vi "Count Digital Pulses Get Date.vi"() -> ()   [LabVIEW 2020]
uses:
  <vilib>/DAQmx/read.llb/DAQmx Read (Counter U32 1Chan 1Samp).vi
  <vilib>/DAQmx/create/channels.llb/DAQmx Create Channel (CI-Count Edges).vi
  <vilib>/DAQmx/miscellaneous.llb/DAQmx Fill In Error Info.vi
panel:
  out "Frequency (Hz)":dbl
  in  "stop":bool
  out "Counts":dbl
  in  "edge":i32(ring)=10280 items=["Rising"=10280, "Falling"=10171]
  in  "count direction":i32(ring)=10128 items=["Count Up"=10128, "Count Down"=10124, "Externally Controlled"=10326]
  in  "initial count":u32
  in  "DAQmx Physical Channel":tag
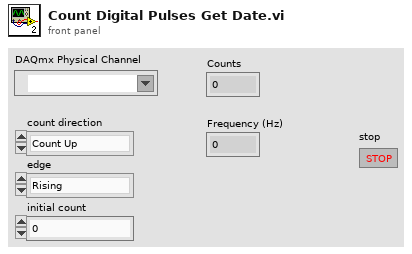
[diagram p1: front panel]
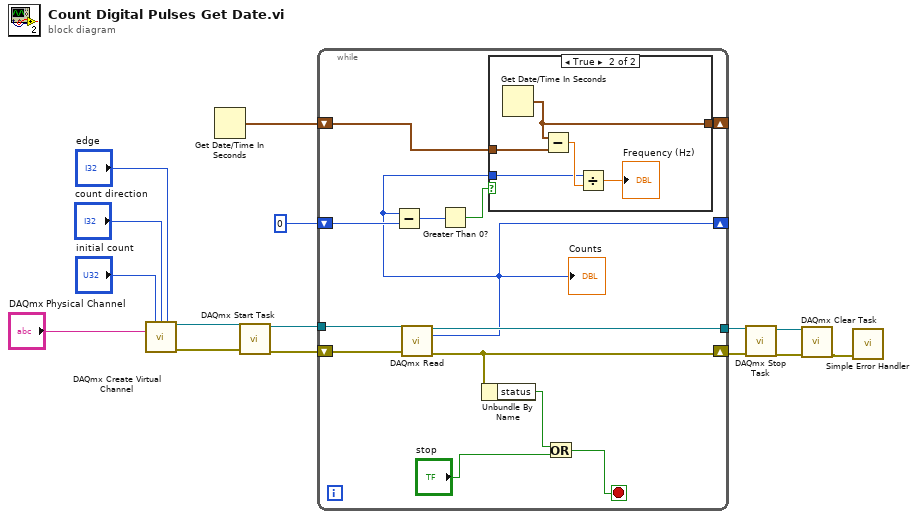
[diagram p0: block diagram]
diagram:
  n1 = call-poly <vilib>:"DAQmx Create Virtual Channel.vi"("initial count"="initial count", "count direction"="count direction", "edge"="edge", "counter"="DAQmx Physical Channel") -> ("task out"=w12:refnum<k21>, "error out"=w11:errorcluster)  [unwired: 10 in]
  n2 = Get Date/Time In Seconds() -> (seconds since 1Jan1904=w1:timestamp)
  n3 = call <vilib>:"DAQmx Start Task.vi"("task/channels in"=w12, "error in"=w11) -> ("task out"=w10:refnum<k21>, "error out"=w9:errorcluster)  [unwired: 12 in]
  n4 = while {
    tunnel: w10 -> [w28]
    tunnel: [w26] -> w8
    shift-right: [w25] -> w7
    shift-left: w9 -> [w27]
    shift-right: [w16] -> _
    shift-left: 0 -> [w21]
    shift-right: [w17] -> _
    shift-left: w1 -> [w18]
    stop <- w22 stop-if-true
    n5 = call-poly <vilib>:"DAQmx Read.vi"("task/channels in"=w28, "error in"=w27) -> ("task out"=w26:refnum<k21>, "data"=w16:u32, "error out"=w25:errorcluster)  [unwired: 11 in]
    "Counts" <- w16
    n6 = Subtract(x=w16, y=w21) -> (x-y=w20:u32)
    n7 = Greater Than 0?(x=w20) -> (x > 0?=w19:bool)
    n8 = Unbundle By Name(w25) -> ("status"=w23:bool)
    n9 = case shown="True" w19 {
      tunnel: w18 -> [w29 w34]
      tunnel: [w29 w33] -> w17
      tunnel: w16 -> [_ w31]
      frame False {
      }
      frame True {
        n10 = Get Date/Time In Seconds() -> (seconds since 1Jan1904=w33:timestamp)
        n11 = Subtract(x=w33, y=w34) -> (x-y=w32:dbl)
        n12 = Divide(x=w31, y=w32) -> (x/y=→"Frequency (Hz)":dbl)
      }
    }
    n13 = Or(x=w23, y="stop") -> (x .or. y?=w22:bool)
  }
  n14 = call <vilib>:"DAQmx Stop Task.vi"("task/channels in"=w8, "error in"=w7) -> ("task out"=w6:refnum<k21>, "error out"=w5:errorcluster)  [unwired: 12 in]
  n15 = call <vilib>:"DAQmx Clear Task.vi"("task in"=w6, "error in"=w5) -> ("error out"=w4:errorcluster)  [unwired: 13 in]
  n16 = call <vilib>:"Simple Error Handler.vi"("error in (no error)"=w4) -> ()  [unwired: 4 in, 5 out]
